vi "EVM_Sweep_Only_R_S_CMP180.vi"() -> ()   [LabVIEW 2023, in "EVM.lvlib"]
uses:
  lib/CTL/LitePoint_EVM_SG.ctl
  lib/CTL/LitePoint_EVM_SA.ctl
  lib/CTL/JIO_FPGA_FTDI.ctl
  EVM.lvlib
  lib/LitePoints/LitePoints.lvlib
  lib/FTDI/JIO/CLC_JIO_FTDI.lvlib
  lib/R_S/R_S.lvlib
panel:
  out "ReceivedPower":dbl format="%#.3g"
  out "Best EVM ALL":dbl
  out "PST(sec)":dbl
  out "Best EVM":dbl
  out "error out":errorcluster
  in  "Power res":i32=2
  in  "Stop Power":i32
  in  "Start Power":i32=-40
  in  "BFIC_ele_stop":i32=12
  in  "BFIC_ele_res":i32=4
  in  "BFIC_ele_start":i32
  in  "BFIC_com_stop":i32=12
  in  "BFIC_com_res":i32=4
  in  "BFIC_com_start":i32
  in  "UD_att_stop":i32=120
  in  "UD_att_res":i32=8
  in  "UD_att_start":i32
  out "UD_att":i32=255
  out "BFIC_com_step":i32=15
  out "BFIC_ele_step":i32=15
  out "SG Power":i32=-10
  in  "TRXmode":u16(ring)=1 items=["Tx"=1, "Rx"=2]
  in  "Polarity":u16(ring) items=["H", "V"]
  out "floder Exist?":bool=TRUE
  in  "Waiting \nTime(ms)":u32=1
  in  "FileNote":string="test16_wayne_MCS11"
  in  "SG":refnum<visa-resource-name>="TCPIP0::192.168.200.50::hislip0::INSTR"
  in  "SA":refnum<visa-resource-name>="TCPIP0::192.168.200.50::hislip0::INSTR"
  out "Spectrum Data":cluster{"X":dbl, "Y":dbl}[](graph)
  # "TMYTEK_CLC_JIO_R&S_EVM_CMP180"
  # "12"
  # "`"
  # "12"
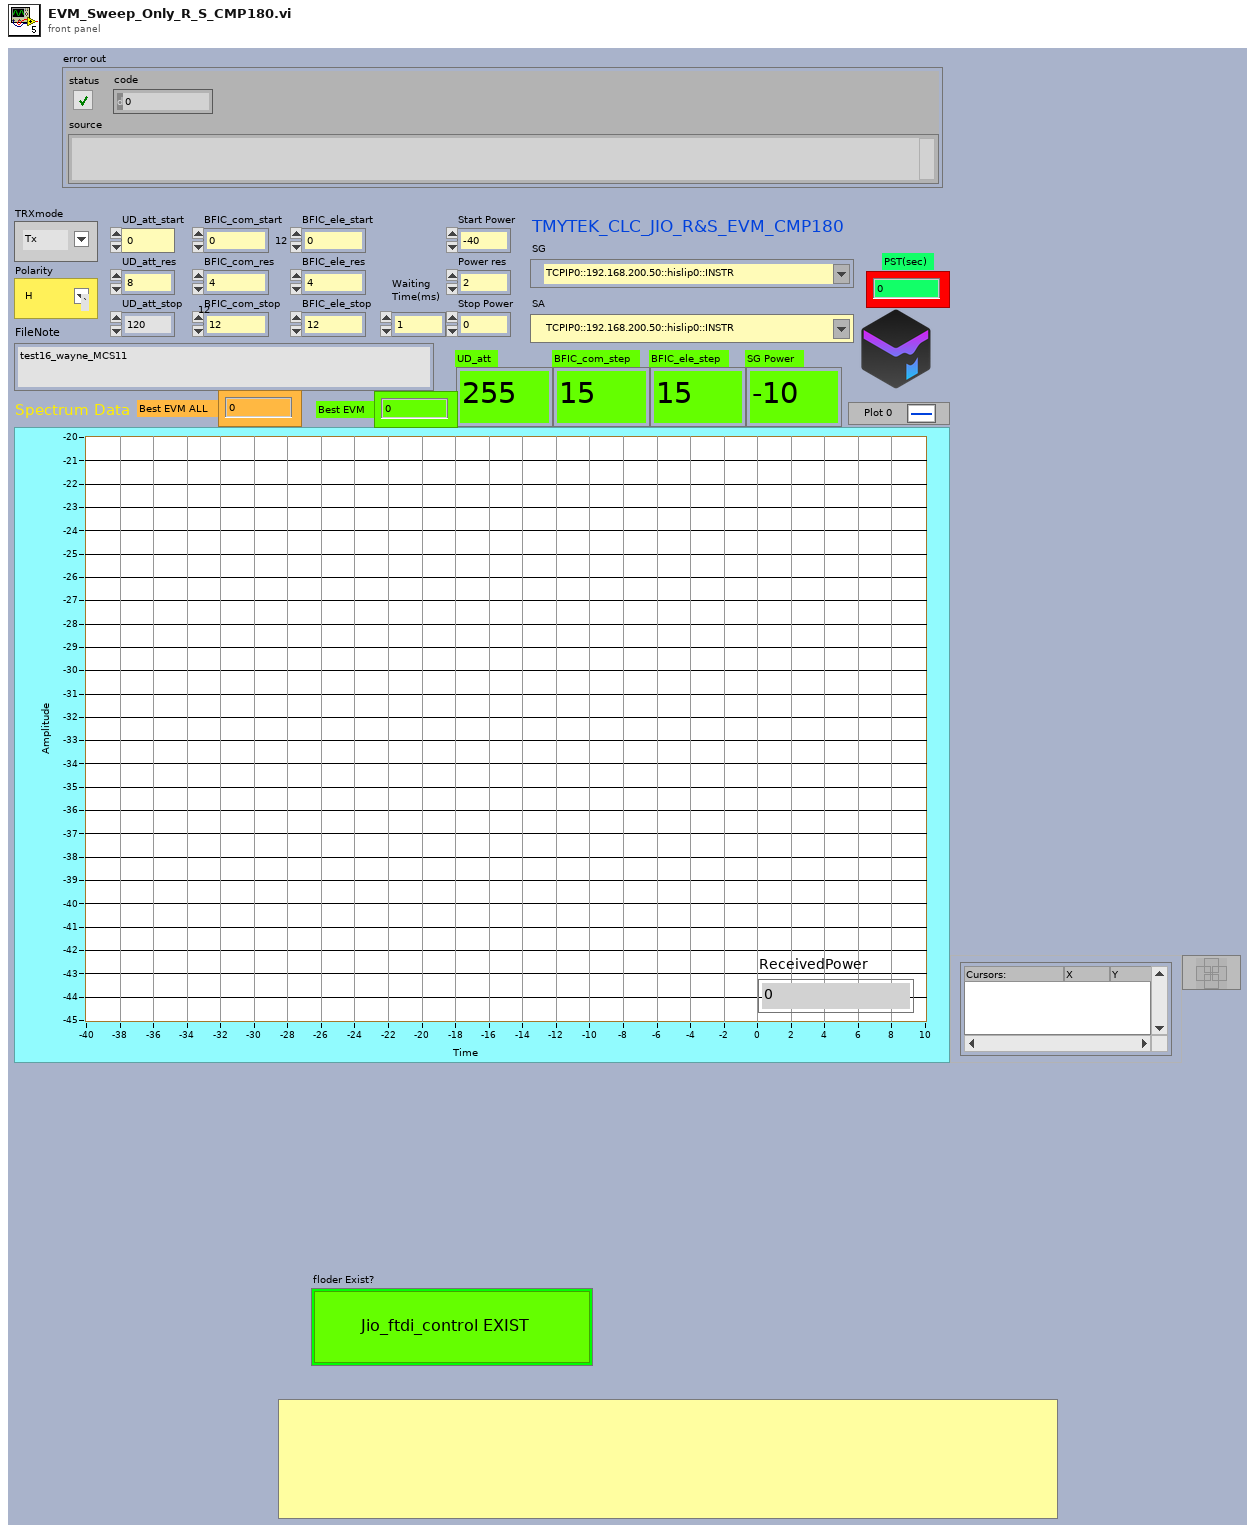
[diagram p1: front panel]
types:
  T1 = typedef "LitePoint_EVM_SG.ctl" = enum16{"Init", "Close", "set_SG", "AdjustLevel", "byPass", "RF_ON", "RF_OFF"}
  T2 = typedef "LitePoint_EVM_SA.ctl" = enum16{"Init", "Close", "set_SA", "get_EVM", "byPass", "getPower"}
  T3 = typedef "JIO_FPGA_FTDI.ctl" = enum16{"Init", "Close", "UD", "BFIC"}
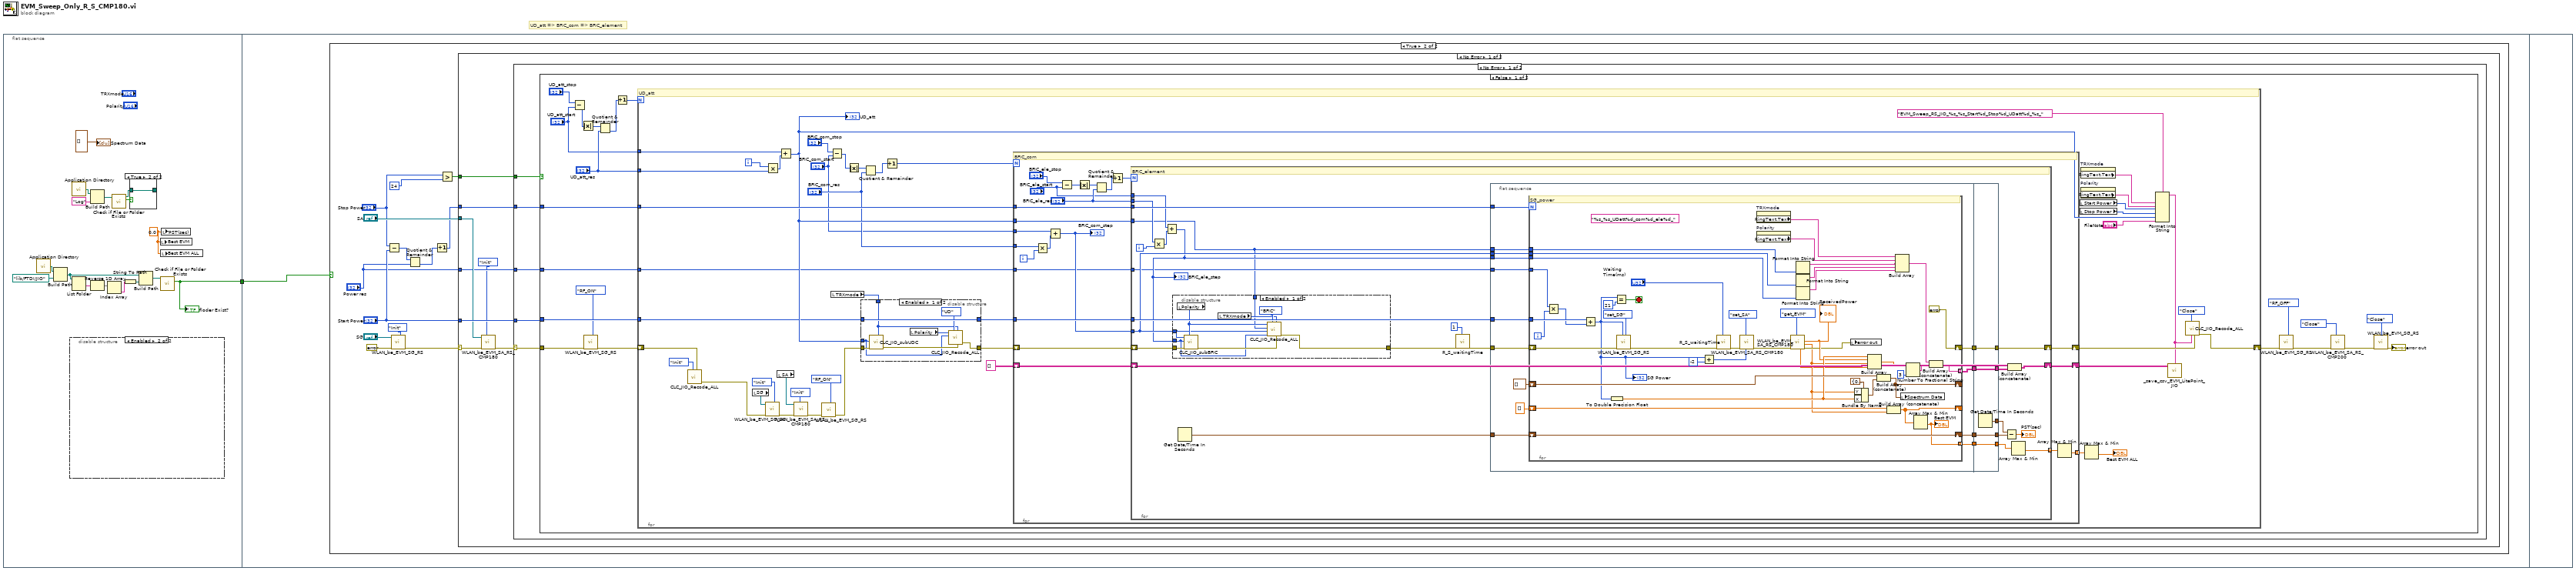
[diagram p0: block diagram]
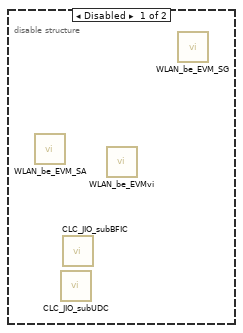
[diagram p2: hidden frame]
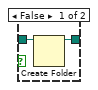
[diagram p3: hidden frame]
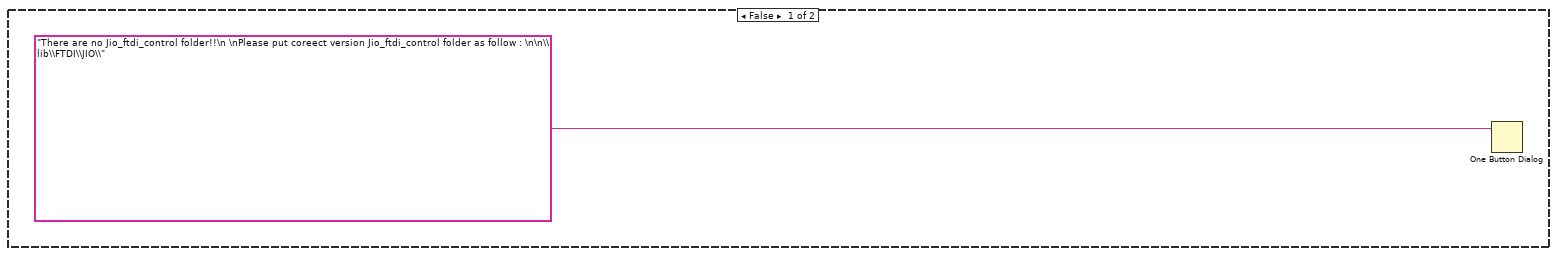
[diagram p4: hidden frame]
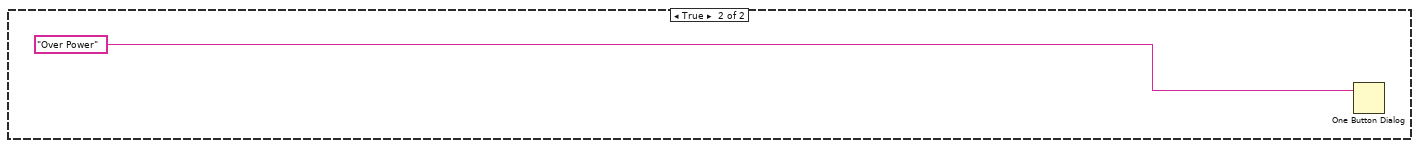
[diagram p7: hidden frame]
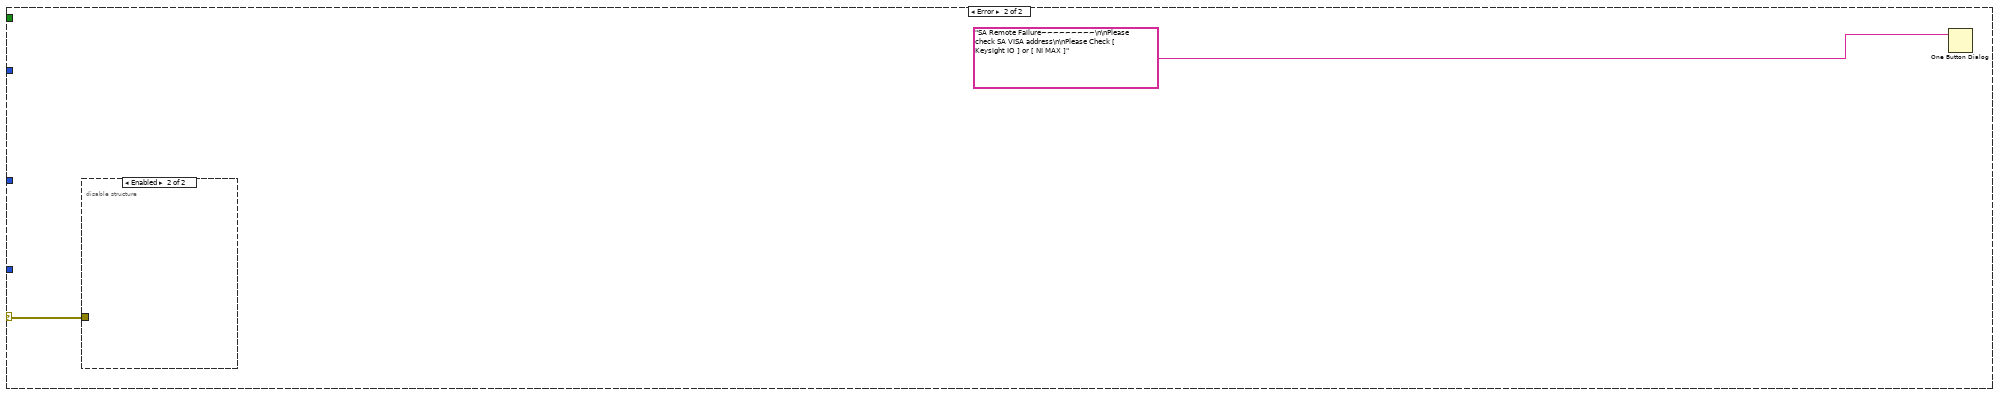
[diagram p8: hidden frame]
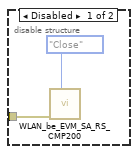
[diagram p9: hidden frame]
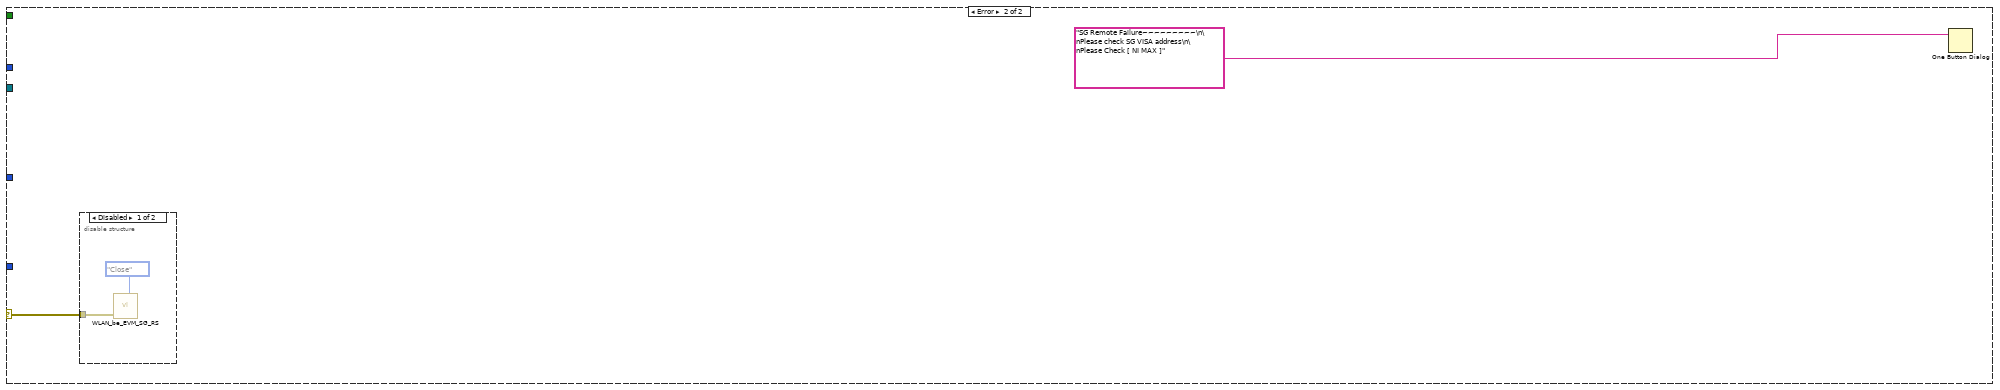
[diagram p10: hidden frame]
diagram:
  # "UD_att => BFIC_com => BFIC_element"
  n1 = flat-sequence {
    tunnel: [w3] -> w1
    tunnel: w1 -> [w21]
    frame #0 {
      w2 = 0.0 ("PST(sec)")
      n2 = call <vilib>:"Application Directory.vi"() -> ("Application Directory"=w9:path)
      n3 = Build Path(base path=w9, name or relative path=path "lib/FTDI/JIO") -> (appended path=w10:path)
      n4 = disable-structure shown="Enabled" {
        frame Disabled {
          n5 = call "WLAN_be_EVM_SA.vi"() -> ()  [unwired: 8 in, 4 out]
          n6 = call "CLC_JIO_subUDC.vi"() -> ()  [unwired: 10 in, 2 out]
          n7 = call "CLC_JIO_subBFIC.vi"() -> ()  [unwired: 10 in, 2 out]
          n8 = call "WLAN_be_EVMvi.vi"() -> ()  [unwired: 8 in, 4 out]
          n9 = call "WLAN_be_EVM_SG.vi"() -> ()  [unwired: 10 in, 2 out]
        }
        frame Enabled {
        }
      }
      n10 = call <vilib>:"Application Directory.vi"() -> ("Application Directory"=w16:path)
      n11 = List Folder(path=w10) -> (folder names=w5:string[])  [unwired: 3 in, 3 out]
      n12 = Reverse 1D Array(array=w5) -> (reversed array=w6:string[])
      n13 = Build Path(base path=w16, name or relative path="Log") -> (appended path=w13:path)
      n14 = Index Array(array=w6) -> (element=w7:string)  [unwired: 1 in]
      n15 = call <vilib>:"Check if File or Folder Exists.vi"("path"=w13) -> ("file or folder exists?"=w15:bool, "dup path"=w14:path)  [unwired: 8 in, 1 out]
      n16 = String To Path(string=w7) -> (path=w8:path)
      n17 = case shown="True" w15 {
        tunnel: w14 -> [w19 w20]
        tunnel: [w18 w20] -> _
        frame False {
          n18 = Create Folder(path (use dialog)=w19) -> (created path=w18:path)  [unwired: 2 in, 2 out]
        }
        frame True {
        }
      }
      n19 = Build Path(base path=w10, name or relative path=w8) -> (appended path=w11:path)
      n20 = local write "Best EVM"(w2) -> ()
      n21 = local write "Best EVM ALL"(w2) -> ()
      n22 = call <vilib>:"Check if File or Folder Exists.vi"("path"=w11) -> ("file or folder exists?"=w3:bool)  [unwired: 8 in, 2 out]
      "floder Exist?" <- w3
      n23 = local write "PST(sec)"(w2) -> ()
      "Spectrum Data" <- cluster{"X":dbl, "Y":dbl}[] [] ("XY Graph")
    }
    frame #1 {
      n24 = case shown="True" w21 {
        frame False {
          n25 = One Button Dialog(message="There are no Jio_ftdi_control folder!!\n \nPlease put coreect version Jio_ftdi_control folder as follow : \n\n\\lib\\FTDI\\JIO\\") -> ()  [unwired: 1 in, 1 out]
        }
        frame True {
          n26 = Subtract(x="Stop Power", y="Start Power") -> (x-y=w26:i32)
          n27 = call "WLAN_be_EVM_SG_RS.vi"("Function_SG"=LitePoint_EVM_SG."Init", "error in"=errorcluster {"status"=FALSE, "code"=0, "source"=""} ("error in (no error)"), "VISA IN"="SG") -> ("error out"=w28:errorcluster)  [unwired: 7 in, 1 out]
          n28 = Quotient & Remainder(x=w26, y="Power res") -> (floor(x/y)=w25:i32)  [unwired: 1 out]
          n29 = Increment(x=w25) -> (x+1=w32:i32)
          n30 = Greater?(x="Stop Power", y=24) -> (0:w34:bool)
          n31 = case shown="No Error" w28 {
            selector: w28 -> [w40 w249]
            tunnel: "SA" -> [w38 _]
            tunnel: w34 -> [w43 _]
            tunnel: "Start Power" -> [w42 _]
            tunnel: w32 -> [w41 _]
            tunnel: "Power res" -> [w37 _]
            frame No Error {
              n32 = call "WLAN_be_EVM_SA_RS_CMP180.vi"("Function"=LitePoint_EVM_SA."Init", "error in"=w40, "VISA IN"=w38) -> ("error out"=w39:errorcluster)  [unwired: 4 in, 4 out]
              n33 = case shown="No Error" w39 {
                selector: w39 -> [w45 w245]
                tunnel: w43 -> [w48 _]
                tunnel: w42 -> [w47 _]
                tunnel: w41 -> [w46 _]
                tunnel: w37 -> [w44 _]
                frame No Error {
                  n34 = case shown="False" w48 {
                    tunnel: w47 -> [w67 _]
                    tunnel: w45 -> [w66 _]
                    tunnel: w46 -> [w68 _]
                    tunnel: w44 -> [w54 _]
                    frame False {
                      n35 = Subtract(x="UD_att_stop", y="UD_att_start") -> (x-y=w61:i32)
                      n36 = Absolute Value(x=w61) -> (abs(x)=w58:i32)
                      n37 = call "WLAN_be_EVM_SG_RS.vi"("Function_SG"=LitePoint_EVM_SG."RF_ON", "error in"=w66) -> ("error out"=w64:errorcluster)  [unwired: 8 in, 1 out]
                      n38 = Quotient & Remainder(x=w58, y="UD_att_res") -> (floor(x/y)=w59:i32)  [unwired: 1 out]
                      n39 = Increment(x=w59) -> (x+1=w55:i32)
                      n40 = for {
                        N: w55 -> [_]
                        tunnel: w68 -> [w111]
                        tunnel: w67 -> [w77]
                        shift-right: [w71] -> w63
                        shift-left: w64 -> [w74]
                        tunnel: "UD_att_res" -> [w98]
                        tunnel: "UD_att_start" -> [w97]
                        tunnel: w54 -> [w88]
                        i -> [w100]
                        # "UD_att"
                        n41 = call "CLC_JIO_Recode_ALL.vi"("error in"=w74, "Function"=JIO_FPGA_FTDI."Init") -> ("error out"=w73:errorcluster)  [unwired: 8 in, 1 out]
                        n42 = local read "SG"() -> (w84:refnum<visa-resource-name>)
                        n43 = call "WLAN_be_EVM_SG_RS.vi"("Function_SG"=LitePoint_EVM_SG."Init", "error in"=w73, "VISA IN"=w84) -> ("error out"=w85:errorcluster)  [unwired: 7 in, 1 out]
                        n44 = Multiply(x=w100, y=w98) -> (x*y=w99:i32)
                        n45 = local read "SA"() -> (w83:refnum<visa-resource-name>)
                        n46 = Add(x=w97, y=w99) -> (x+y=w96:i32)
                        "UD_att" <- w96
                        n47 = call "WLAN_be_EVM_SA_RS_CMP180.vi"("Function"=LitePoint_EVM_SA."Init", "error in"=w85, "VISA IN"=w83) -> ("error out"=w81:errorcluster)  [unwired: 4 in, 4 out]
                        n48 = call "WLAN_be_EVM_SG_RS.vi"("Function_SG"=LitePoint_EVM_SG."RF_ON", "error in"=w81) -> ("error out"=w80:errorcluster)  [unwired: 8 in, 1 out]
                        n49 = Subtract(x="BFIC_com_stop", y="BFIC_com_start") -> (x-y=w95:i32)
                        n50 = local read "TRXmode"() -> (w108:u16)
                        n51 = Absolute Value(x=w95) -> (abs(x)=w94:i32)
                        n52 = disable-structure shown="Enabled" {
                          disable-tunnel: [w117 w120] -> w110
                          disable-tunnel: w80 -> [w119 w120]
                          disable-tunnel: w108 -> [w114 _]
                          disable-tunnel: w96 -> [w112 _]
                          disable-tunnel: [w116 _] -> w76
                          disable-tunnel: w77 -> [w116 _]
                          frame Enabled {
                            n53 = call "CLC_JIO_subUDC.vi"("Mode"=w114, "error in"=w119, "ud att"=w112) -> ("error out"=w118:errorcluster)  [unwired: 7 in, 1 out]
                            n54 = local read "Polarity"() -> (w113:u16)
                            n55 = call "CLC_JIO_Recode_ALL.vi"("error in"=w118, "Mode"=w114, "Function"=JIO_FPGA_FTDI."UD", "UD_att"=w112, "pol"=w113) -> ("error out"=w117:errorcluster)  [unwired: 5 in, 1 out]
                          }
                          frame Disabled {
                          }
                        }
                        n56 = Quotient & Remainder(x=w94, y="BFIC_com_res") -> (floor(x/y)=w90:i32)  [unwired: 1 out]
                        n57 = Increment(x=w90) -> (x+1=w89:i32)
                        n58 = for {
                          N: w89 -> [_]
                          tunnel: w111 -> [w142]
                          tunnel: w76 -> [w141]
                          shift-right: [w138] -> w109
                          shift-left: string[][] [] -> [w139]
                          tunnel: w96 -> [w137]
                          shift-right: [w136] -> w72
                          shift-left: w110 -> [w140]
                          tunnel: "BFIC_com_res" -> [w132]
                          tunnel: "BFIC_com_start" -> [w131]
                          tunnel: w88 -> [w123]
                          tunnel: [w121] -> w79 mode=indexing
                          i -> [w134]
                          # "BFIC_com"
                          n59 = Multiply(x=w132, y=w134) -> (x*y=w135:i32)
                          n60 = Add(x=w131, y=w135) -> (x+y=w133:i32)
                          "BFIC_com_step" <- w133
                          n61 = Subtract(x="BFIC_ele_stop", y="BFIC_ele_start") -> (x-y=w129:i32)
                          n62 = Absolute Value(x=w129) -> (abs(x)=w130:i32)
                          n63 = Quotient & Remainder(x=w130, y="BFIC_ele_res") -> (floor(x/y)=w127:i32)  [unwired: 1 out]
                          n64 = Increment(x=w127) -> (x+1=w124:i32)
                          n65 = for {
                            N: w124 -> [_]
                            tunnel: w142 -> [w170]
                            tunnel: w141 -> [w169]
                            shift-right: [w167] -> w138
                            shift-left: w139 -> [w166]
                            tunnel: w133 -> [w162]
                            tunnel: w137 -> [w143]
                            shift-right: [w147] -> w136
                            shift-left: w140 -> [w165]
                            tunnel: "BFIC_ele_res" -> [w158]
                            tunnel: "BFIC_ele_start" -> [w157]
                            tunnel: w123 -> [w156]
                            tunnel: [w144] -> w122 mode=indexing
                            i -> [w159]
                            # "BFIC_element"
                            n66 = Multiply(x=w158, y=w159) -> (x*y=w161:i32)
                            n67 = Add(x=w157, y=w161) -> (x+y=w160:i32)
                            "BFIC_ele_step" <- w160
                            n68 = disable-structure shown="Enabled" {
                              disable-tunnel: w165 -> [w242 w243]
                              disable-tunnel: [w240 w243] -> w164
                              disable-tunnel: w160 -> [w234 _]
                              disable-tunnel: w162 -> [w235 _]
                              disable-tunnel: w143 -> [w236 _]
                              frame Enabled {
                                n69 = local read "Polarity"() -> (w237:u16)
                                n70 = call "CLC_JIO_subBFIC.vi"("pol"=w237, "error in"=w242, "ele"=w234, "com"=w235) -> ("error out"=w241:errorcluster)  [unwired: 6 in, 1 out]
                                n71 = local read "TRXmode"() -> (w238:u16)
                                n72 = call "CLC_JIO_Recode_ALL.vi"("error in"=w241, "Mode"=w238, "Function"=JIO_FPGA_FTDI."BFIC", "ele_att"=w234, "com_att"=w235, "UD_att"=w236, "pol"=w237) -> ("error out"=w240:errorcluster)  [unwired: 3 in, 1 out]
                              }
                              frame Disabled {
                              }
                            }
                            n73 = Get Date/Time In Seconds() -> (seconds since 1Jan1904=w154:timestamp)
                            n74 = call "R_S_waitingTime.vi"("Waiting Time(ms)"=u32 1, "error in"=w164) -> ("error out"=w155:errorcluster)  [unwired: 9 in]
                            n75 = flat-sequence {
                              tunnel: w170 -> [w184]
                              tunnel: w169 -> [w182]
                              tunnel: w143 -> [w180]
                              tunnel: w162 -> [w179]
                              tunnel: w160 -> [w177]
                              tunnel: w156 -> [w176]
                              tunnel: w155 -> [w175]
                              tunnel: w154 -> [w173]
                              tunnel: [w181] -> w152
                              tunnel: [w178] -> w151
                              tunnel: [w172] -> w150
                              tunnel: [w171] -> w146
                              tunnel: [w231] -> w153
                              tunnel: [w232] -> w147
                              tunnel: [w233] -> w168
                              tunnel: w152 -> [w233]
                              tunnel: w151 -> [w232]
                              tunnel: w150 -> [w231]
                              tunnel: [w230] -> w149
                              tunnel: [w229] -> w145
                              tunnel: w146 -> [w229]
                              frame #0 {
                                n76 = for {
                                N: w184 -> [_]
                                tunnel: w182 -> [w228]
                                shift-right: [errorcluster {"status"=FALSE, "code"=0, "source"=""} ("error out")] -> w178
                                shift-left: w175 -> [w220]
                                shift-right: [w222] -> _
                                shift-left: cluster{"X":dbl, "Y":dbl}[] [] ("XY Graph") -> [w224]
                                tunnel: [w212] -> w181 mode=indexing
                                tunnel: w180 -> [w209]
                                tunnel: w177 -> [w207]
                                tunnel: w179 -> [w208]
                                tunnel: w176 -> [w201]
                                shift-right: [w189] -> _
                                shift-left: dbl[] [] -> [w191]
                                shift-right: [w188] -> w172
                                shift-left: w173 -> [w188]
                                tunnel: [w186] -> w171 mode=indexing
                                i -> [w202]
                                stop <- w226 stop-if-true
                                (unwired) "%s_%s_UDatt%d_com%d_ele%d_" ("format string")
                                # "SG_power"
                                n77 = Multiply(x=w201, y=w202) -> (x*y=w200:i32)
                                n78 = Add(x=w228, y=w200) -> (x+y=w194:i32)
                                "SG Power" <- w194
                                n79 = To Double Precision Float(number=w194) -> (double precision float=w221:dbl)
                                n80 = Equal?(x=w194, y=21) -> (x = y?=w226:bool)
                                n81 = call "WLAN_be_EVM_SG_RS.vi"("Function_SG"=LitePoint_EVM_SG."set_SG", "setPower"=w194, "error in"=w220) -> ("error out"=w198:errorcluster)  [unwired: 7 in, 1 out]
                                n82 = Add(x=w194, y=-2) -> (x+y=w193:i32)
                                n83 = call "R_S_waitingTime.vi"("Waiting Time(ms)"="Waiting \nTime(ms)", "error in"=w198) -> ("error out"=w216:errorcluster)  [unwired: 9 in]
                                n84 = call "WLAN_be_EVM_SA_RS_CMP180.vi"("SG Power"=w193, "Function"=LitePoint_EVM_SA."set_SA", "error in"=w216) -> ("error out"=w196:errorcluster)  [unwired: 4 in, 4 out]
                                n85 = property on="TRXmode" class="Ring (strict)"() -> ("RingText.Text"=w211:string)  [unwired: 2 in, 2 out]
                                n86 = property on="Polarity" class="Ring (strict)"() -> ("RingText.Text"=w210:string)  [unwired: 2 in, 2 out]
                                n87 = call "WLAN_be_EVM_SA_RS_CMP180.vi"("Function"=LitePoint_EVM_SA."get_EVM", "error in"=w196) -> ("error out"=w195:errorcluster, "EVM"=w190:dbl, "Power"=w199:dbl, "FreqError"=w185:dbl)  [unwired: 5 in, 1 out]
                                "ReceivedPower" <- w199
                                n88 = Format Into String(w209) -> (resulting string=w206:string)  [unwired: 3 in, 1 out]
                                n89 = Format Into String(w208) -> (resulting string=w205:string)  [unwired: 3 in, 1 out]
                                n90 = Format Into String(w207) -> (resulting string=w204:string)  [unwired: 3 in, 1 out]
                                n91 = local write "error out"(w195) -> ()
                                n92 = Bundle By Name(cluster=cluster{"X":dbl, "Y":dbl} {"X"=0.0, "Y"=0.0} ("element"), "Y"=w190, "X"=w221) -> (w223:cluster{"X":dbl, "Y":dbl})
                                n93 = Build Array(w221, w199, w190, w185) -> (w214:dbl[])
                                n94 = Build Array (concatenate)(w224, w223) -> (w222:cluster{"X":dbl, "Y":dbl}[])
                                n95 = Build Array (concatenate)(w191, w190) -> (w189:dbl[])
                                n96 = Build Array(w211, w210, w206, w205, w204) -> (w203:string[])
                                n97 = local write "Spectrum Data"(w222) -> ()
                                n98 = Number To Fractional String(number=w214, precision (6)=i16 3) -> (F-format string=w213:string[])  [unwired: 2 in]
                                n99 = Array Max & Min(array=w189) -> (min value=w186:dbl)  [unwired: 3 out]
                                "Best EVM" <- w186
                                n100 = Build Array (concatenate)(w203, w213) -> (w212:string[])
                                }
                              }
                              frame #1 {
                                n101 = Get Date/Time In Seconds() -> (seconds since 1Jan1904=w230:timestamp)
                              }
                            }
                            n102 = Subtract(x=w149, y=w153) -> (x-y=→"PST(sec)":dbl)
                            n103 = Build Array (concatenate)(w166, w168) -> (w167:string[][])
                            n104 = Array Max & Min(array=w145) -> (min value=w144:dbl)  [unwired: 3 out]
                          }
                          n105 = Array Max & Min(array=w122) -> (min value=w121:dbl)  [unwired: 3 out]
                        }
                        n106 = local read "Start Power"() -> (w104:i32)
                        n107 = local read "Stop Power"() -> (w106:i32)
                        n108 = property on="TRXmode" class="Ring (strict)"() -> ("RingText.Text"=w102:string)  [unwired: 2 in, 2 out]
                        n109 = property on="Polarity" class="Ring (strict)"() -> ("RingText.Text"=w103:string)  [unwired: 2 in, 2 out]
                        n110 = Array Max & Min(array=w79) -> (min value=→"Best EVM ALL":dbl)  [unwired: 3 out]
                        n111 = Format Into String(format string="EVM_Sweep_RS_JIO_%s_%s_Start%d_Stop%d_UDatt%d_%s_" ("delimiter (\\t)"), w102, w103, w104, w106, w96, "FileNote") -> (resulting string=w69:string)  [unwired: 2 in, 1 out]
                        n112 = call "_save_csv_EVM_LitePoint_JIO.vi"("delimiter (\\t)"=w69, "array in"=w109) -> ()  [unwired: 9 in, 1 out]
                        n113 = call "CLC_JIO_Recode_ALL.vi"("error in"=w72, "FileName"=w69, "Function"=JIO_FPGA_FTDI."Close") -> ("error out"=w71:errorcluster)  [unwired: 7 in, 1 out]
                      }
                      n114 = call "WLAN_be_EVM_SG_RS.vi"("Function_SG"=LitePoint_EVM_SG."RF_OFF", "error in"=w63) -> ("error out"=w51:errorcluster)  [unwired: 8 in, 1 out]
                      n115 = call "WLAN_be_EVM_SA_RS_CMP200.vi"("Function"=LitePoint_EVM_SA."Close", "error in"=w51) -> ("error out"=w50:errorcluster)  [unwired: 6 in, 3 out]
                      n116 = call "WLAN_be_EVM_SG_RS.vi"("Function_SG"=LitePoint_EVM_SG."Close", "error in"=w50) -> ("error out"=→"error out":errorcluster)  [unwired: 8 in, 1 out]
                    }
                    frame True {
                      n117 = One Button Dialog(message="Over Power") -> ()  [unwired: 1 in, 1 out]
                    }
                  }
                }
                frame Error {
                  n118 = disable-structure shown="Enabled" {
                    disable-tunnel: w245 -> [w248 _]
                    frame Disabled {
                      n119 = call "WLAN_be_EVM_SA_RS_CMP200.vi"("Function"=LitePoint_EVM_SA."Close", "error in"=w248) -> ()  [unwired: 6 in, 4 out]
                    }
                    frame Enabled {
                    }
                  }
                  n120 = One Button Dialog(message="SA Remote Failure~~~~~~~~~\n\nPlease check SA VISA address\n\nPlease Check [ Keysight IO ] or [ NI MAX ]") -> ()  [unwired: 1 in, 1 out]
                }
              }
            }
            frame Error {
              n121 = disable-structure shown="Disabled" {
                disable-tunnel: w249 -> [w252 _]
                frame Disabled {
                  n122 = call "WLAN_be_EVM_SG_RS.vi"("Function_SG"=LitePoint_EVM_SG."Close", "error in"=w252) -> ()  [unwired: 8 in, 2 out]
                }
                frame Enabled {
                }
              }
              n123 = One Button Dialog(message="SG Remote Failure~~~~~~~~~\n\nPlease check SG VISA address\n\nPlease Check [ NI MAX ]") -> ()  [unwired: 1 in, 1 out]
            }
          }
        }
      }
    }
    frame #2 {
    }
  }
